vi "Open Session (Poly).vi"   [LabVIEW 2014, in "niHighSpeedSerial Eye Scan v1 Host.lvclass"]
doc: "Opens an Eye Scan session with the specified parameters."
uses:
  <instrlib>/niHighSpeedSerial/Eye Scan/v1/Host/Eye Scan/niHighSpeedSerial Eye Scan v1 Host.lvclass
  <instrlib>/niHighSpeedSerial/Eye Scan/v1/Host/Impl/N Point Eye Scan/niHighSpeedSerial N Point Eye Scan v1 Host.lvclass
  <instrlib>/niHighSpeedSerial/Eye Scan/v1/Host/Impl/Rectangular Eye Scan/niHighSpeedSerial Rectangular Eye Scan v1 Host.lvclass
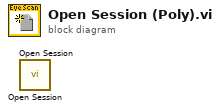
[diagram p0: block diagram]
diagram:
  n1 = call <instrlib>:"Open Session.vi"() -> ()  [unwired: 14 in, 2 out]
  n2 = call <instrlib>:"Open Session.vi"() -> ()  [unwired: 14 in, 2 out]
